vi "PicoScope2000 - Fast Streaming -PM.vi"() -> ()   [LabVIEW 2017]
uses:
  PicoScope2000.llb/GlobalStop.vi
  PS2000.dll
  Program Files (x86)/Pico Technology/SDK/lib/ps2000Wrap.dll
panel:
  out "Post capture information":T1
  out "Previous Total":u32
  out "Number of Samples":u32
  out "Channel A - Post capture raw data":i16[](graph)
  out "Channel A - Live":i16[](graph)
  out "Total Samples":u32
  out "Auto Stopped":bool
  out "Application Buffer Full":bool
  out "overflow":i16
  out "Trigger":cluster{bool, "triggeredAt  Index (Total)":u32}
  out "Sample Interval":u32
  in  "stop":bool
  in  "Acquisition Settings":T2={"Auto Stop"=TRUE, "Desired Sample Interval"=1, "Max Samples"=2000000, "Num Samples per Aggregate"=1, "Overview Buffer Size"=200000, "Time Units"=3, "Application Buffer Size"=25000000} {"Time Units" items=["Nanoseconds (ns)"=2, "Microseconds (us)"=3, "Milliseconds (ms)"=4, "Seconds (s)"=5]}
  in  "Channel A Settings":T3={"Enabled"=TRUE, "Coupling"=1, "Range"=6} {"Range" items=["10 mV", "20 mV", "50 mV", "100 mV", "200 mV", "500 mV", "1 V", "2 V", "5 V", "10 V", "20 V", "50 V ", "100 V"]; "Coupling" items=["AC", "DC"]}
  in  "Channel B Settings":T3={"Enabled"=FALSE, "Coupling"=1, "Range"=6} {"Range" items=["10 mV", "20 mV", "50 mV", "100 mV", "200 mV", "500 mV", "1 V", "2 V", "5 V", "10 V", "20 V", "50 V ", "100 V"]; "Coupling" items=["AC", "DC"]}
  in  "Trigger Settings":T4={"Trigger Enabled"=TRUE, "Trigger Source"=enum."Channel A", "Trigger Threshold (mV)"=500, "Trigger Direction"=2, "Trigger Delay (%)"=0, "Auto Trigger Time (ms)"=0} {"Trigger Direction" items=["Rising"=2, "Falling"=3]}
  # "NOTE: This chart is for indication purposes only - retrieve data values from the app buffer or driver post capture."
  # "Triggered"
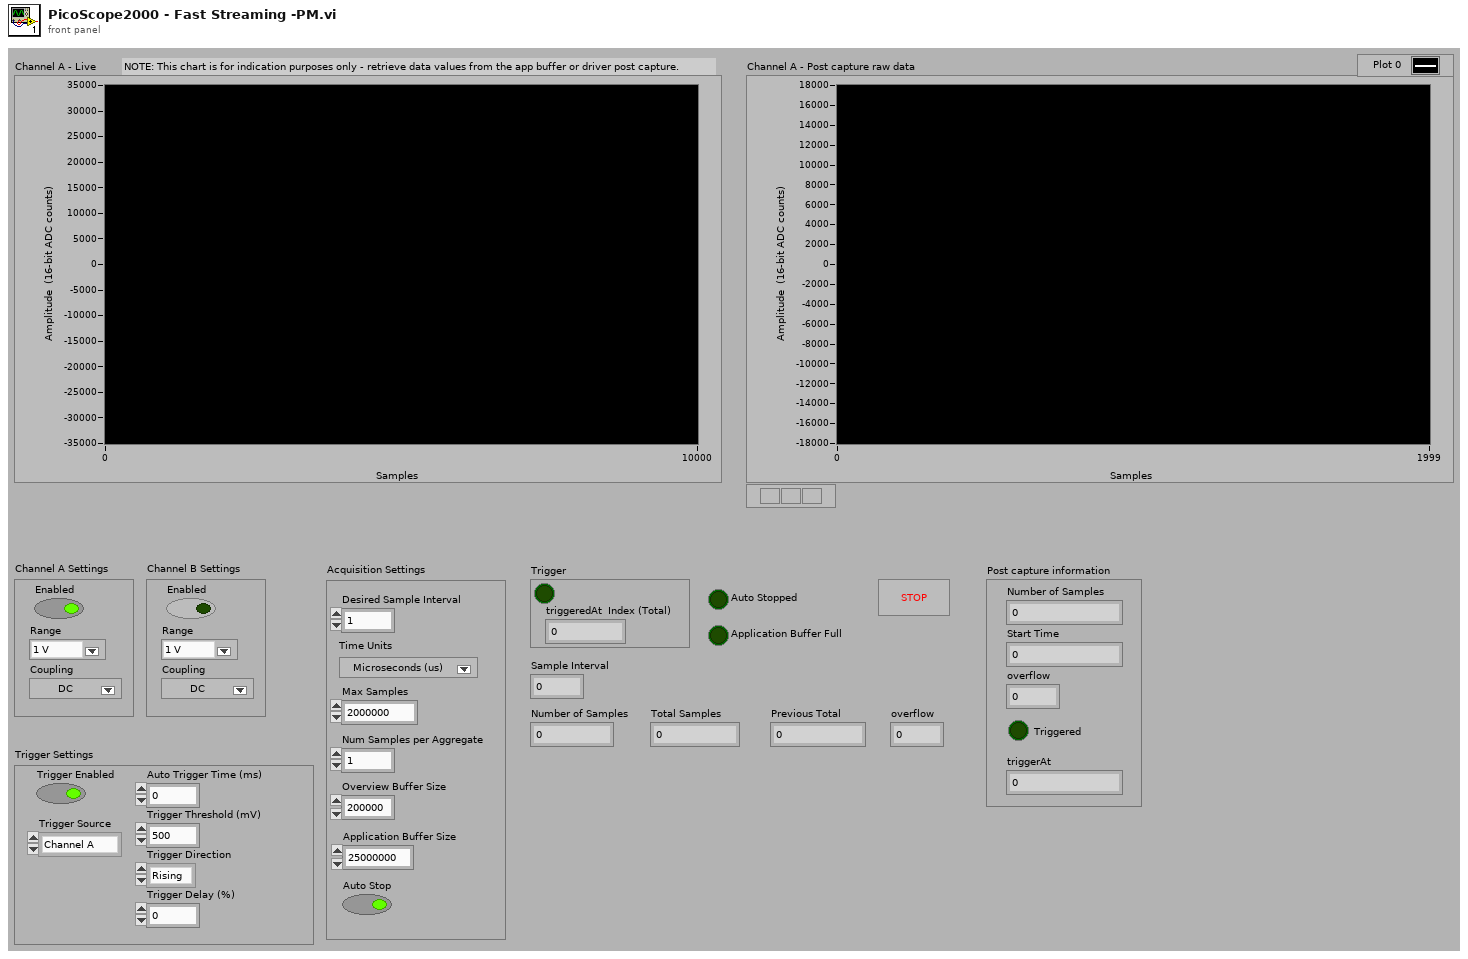
[diagram p1: front panel]
types:
  T1 = cluster{"Number of Samples":u32, "Start Time":dbl, "overflow":i16, bool, "triggerAt":u32}
  T2 = cluster{"Auto Stop":bool, "Desired Sample Interval":u32, "Max Samples":u32, "Num Samples per Aggregate":u32, "Overview Buffer Size":u32, "Time Units":u32, "Application Buffer Size":u32}
  T3 = cluster{"Enabled":bool, "Coupling":i16, "Range":u16}
  T4 = cluster{"Trigger Enabled":bool, "Trigger Source":enum16{"Channel A", "Channel B", "Channel C", "Channel D", "Ext."}, "Trigger Threshold (mV)":i16, "Trigger Direction":i16, "Trigger Delay (%)":i16, "Auto Trigger Time (ms)":i16}
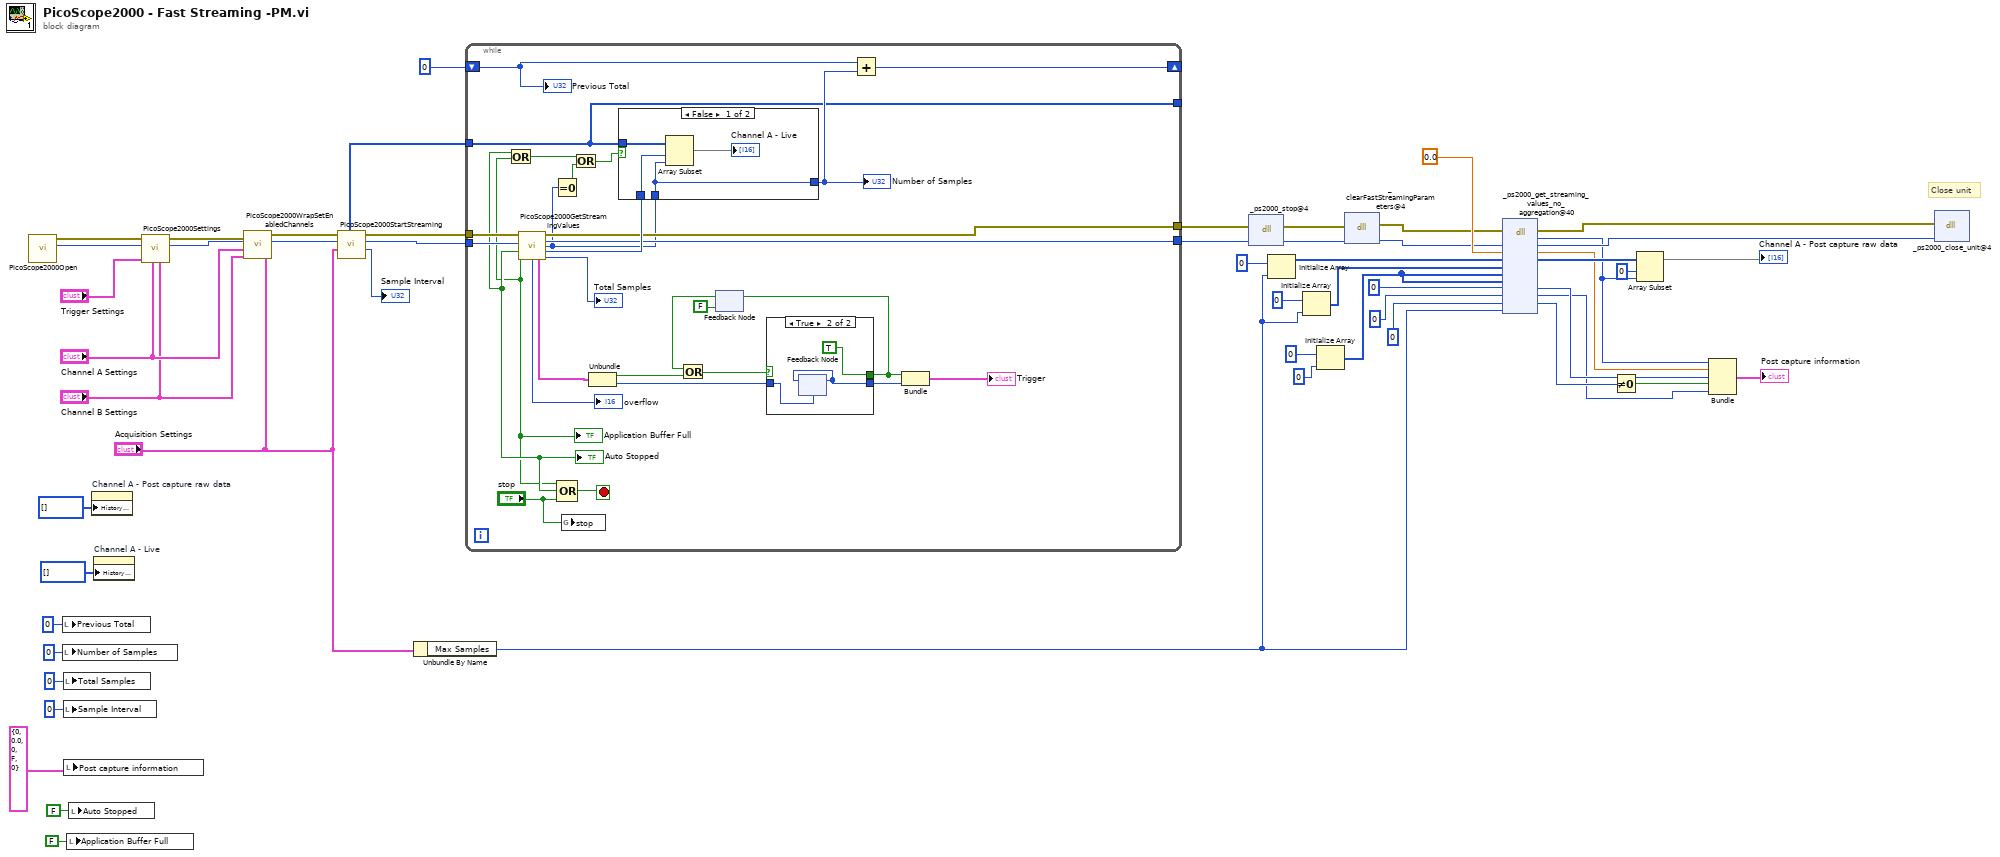
[diagram p0: block diagram]
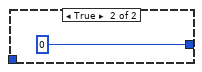
[diagram p2: hidden frame]
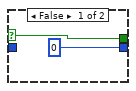
[diagram p3: hidden frame]
diagram:
  # "Close unit"
  n1 = call "PicoScope2000Open.vi"() -> ("handle"=w53:i16, "error out"=w54:errorcluster)  [unwired: 8 in]
  n2 = local write "Previous Total"(u32 0 ("Previous Total")) -> ()
  n3 = local write "Number of Samples"(u32 0 ("Number of Samples")) -> ()
  n4 = local write "Total Samples"(u32 0 ("Total Samples")) -> ()
  n5 = local write "Sample Interval"(u32 0 ("Sample Interval")) -> ()
  n6 = local write "Post capture information"(T1 {"Number of Samples"=0, "Start Time"=0.0, "overflow"=0, FALSE, "triggerAt"=0} ("Post capture information")) -> ()
  n7 = local write "Application Buffer Full"(FALSE ("Application Buffer Full")) -> ()
  n8 = local write "Auto Stopped"(FALSE ("Auto Stopped")) -> ()
  n9 = property on="Channel A - Post capture raw data" class="WFChart (strict)"("History Data"=i16[] []) -> ()  [unwired: 2 in, 2 out]
  n10 = property on="Channel A - Live" class="WFChart (strict)"("History Data"=i16[] []) -> ()  [unwired: 2 in, 2 out]
  n11 = call "PicoScope2000Settings.vi"("Channel B Settings"="Channel B Settings", "Channel A Settings"="Channel A Settings", "Trigger Settings"="Trigger Settings", "handle in"=w53, "error in"=w54) -> ("handle out"=w5:i16, "error out"=w51:errorcluster)  [unwired: 3 in]
  n12 = call "PicoScope2000WrapSetEnabledChannels.vi"("Acquisition Settings"="Acquisition Settings", "Channel B Settings"="Channel B Settings", "Channel A Settings"="Channel A Settings", "handle in"=w5, "error in (no error)"=w51) -> ("handle out"=w4:i16, "error out"=w50:errorcluster)  [unwired: 1 in]
  n13 = call "PicoScope2000StartStreaming.vi"("Acquisition Settings"="Acquisition Settings", "handle in"=w4, "error in"=w50) -> ("Sample Interval"=→"Sample Interval":u32, "handle out"=w48:i16, "error out"=w49:errorcluster, "Channel A"=w47:i16[])  [unwired: 2 in, 1 out]
  n14 = Unbundle By Name("Acquisition Settings") -> ("Max Samples"=w24:u32)
  n15 = while {
    tunnel: w49 -> [w82]
    tunnel: w48 -> [w81]
    tunnel: w47 -> [w56]
    tunnel: [w78] -> w46
    tunnel: [w76] -> w45
    shift-right: [w65] -> _
    shift-left: u32 0 -> [w64]
    tunnel: [w56] -> _
    stop <- w77 stop-if-true
    n16 = call "PicoScope2000GetStreamingValues.vi"("error in"=w82, "handle in"=w81) -> ("error out"=w76:errorcluster, "handle out"=w78:i16, "Number of Samples"=w57:u32, "Auto Stopped"=w62:bool, "App Buffer startIndex"=w79:u32, "Application Buffer Full"=w61:bool, "overflow"=→"overflow":i16, "Trigger"=w74:cluster{bool, "triggeredAt  Index (Total)":u32}, "Total Samples"=→"Total Samples":u32)  [unwired: 5 in]
    "Application Buffer Full" <- w61
    "Auto Stopped" <- w62
    n17 = Or(x=w62, y=w61) -> (x .or. y?=w60:bool)
    n18 = Equal To 0?(x=w57) -> (x = 0?=w58:bool)
    n19 = Compound Arithmetic op=OR(w61, w62, "stop") -> (w77:bool)
    n20 = global write "GlobalStop.vi" "stop"("stop") -> ()
    n21 = Or(x=w60, y=w58) -> (x .or. y?=w59:bool)
    n22 = Unbundle(w74) -> (w67:bool, "triggeredAt  Index (Total)"=w72:u32)
    n23 = case shown="False" w59 {
      tunnel: w79 -> [w86 _]
      tunnel: w56 -> [w85 _]
      tunnel: w57 -> [w84 _]
      tunnel: [w84 u32 0 ("Number of Samples")] -> w63
      frame False {
        n24 = Array Subset(array=w85, index=w86, length=w84) -> (→"Channel A - Live":i16[])
      }
      frame True {
      }
    }
    "Number of Samples" <- w63
    n25 = feedback #1(FALSE) -> (w68:bool)
    n26 = Or(x=w68, y=w67) -> (x .or. y?=w69:bool)
    n27 = case shown="True" w69 {
      selector: w69 -> [w89 _]
      tunnel: w72 -> [_ w92]
      tunnel: [u32 0 ("triggeredAt  Index (Total)") w91] -> w71
      tunnel: [w89 TRUE] -> w70
      frame False {
      }
      frame True {
        n28 = feedback #2(w92) -> (w91:u32)
        n29 = feedback-in #2(w91) -> ()
      }
    }
    n30 = feedback-in #1(w70) -> ()
    n31 = Add(x=w64, y=w63) -> (x+y=w65:u32)
    n32 = Bundle(w70, "triggeredAt  Index (Total)"=w71) -> (→"Trigger":cluster{bool, "triggeredAt  Index (Total)":u32})  [unwired: 1 in]
    "Previous Total" <- w64
  }
  n33 = dll-call lib="PS2000.dll" fn="_ps2000_stop@4" label="ps2000_stop"(error in=w45, "handle"=w46) -> (error out=w44:errorcluster, "handle"=w41:i16)  [unwired: 3 in, 1 out]
  n34 = Initialize Array(i16 0 ("triggerAt"), w24) -> (w33:i16[])
  n35 = Initialize Array(i16 0 ("triggerAt"), w24) -> (w29:i16[])
  n36 = Initialize Array(i16 0 ("triggerAt"), u32 0 ("triggerAt")) -> (w28:i16[])
  n37 = dll-call lib="C:/Program Files (x86)/Pico Technology/SDK/lib/ps2000Wrap.dll" fn="_clearFastStreamingParameters@4" label="clearFastStreamingParameters"(error in=w44, "handle"=w41) -> (error out=w35:errorcluster, "handle"=w37:i16)  [unwired: 3 in, 1 out]
  n38 = dll-call lib="ps2000.dll" fn="_ps2000_get_streaming_values_no_aggregation@40" label="ps2000_get_streaming_values_no_aggregation"(error in=w35, "handle"=w37, "Start Time"=0.0 ("start_time"), "buffer_a"=w33, "buffer_b"=w29, "buffer_c"=w28, "buffer_d"=w28, "overflow"=i16 0 ("triggerAt"), "triggerAt"=u32 0 ("number"), "trigger"=i16 0, "no_of_values"=w24) -> (error out=w6:errorcluster, "Number of Samples"=w21:u32, "handle"=w36:i16, "Start Time"=w20:dbl, "buffer_a"=w26:i16[], "overflow"=w15:i16, "triggerAt"=w13:u32, "trigger"=w19:i16)  [unwired: 6 in, 1 out]
  n39 = Not Equal To 0?(x=w19) -> (x != 0?=w14:bool)
  n40 = Array Subset(array=w26, index=0, length=w21) -> (→"Channel A - Post capture raw data":i16[])
  n41 = Bundle("Number of Samples"=w21, "Start Time"=w20, "overflow"=w15, w14, "triggerAt"=w13) -> (→"Post capture information":T1)  [unwired: 1 in]
  n42 = dll-call lib="PS2000.dll" fn="_ps2000_close_unit@4"(error in=w6, "handle"=w36) -> ()  [unwired: 4 in, 2 out]
